vi "Replace Array Subset (Multi).vi"(5 "JSON Array":refnum<class "JSON Array.lvclass">, 9 "index":i32, 11 "new element/subarray":refnum<class "JSON Null.lvclass">[](array[class])) -> (6 "output JSON Array":refnum<class "JSON Array.lvclass">)   [LabVIEW 2016, in "LVJSON.lvlib" / "JSON Array.lvclass"]
doc: "Replaces an element or subarray in an array at the point you specify in index."
uses:
  JSON Array.lvclass
  JSON Datatype/JSON Null.lvclass
  JSON Array.lvclass/JSON Array.ctl
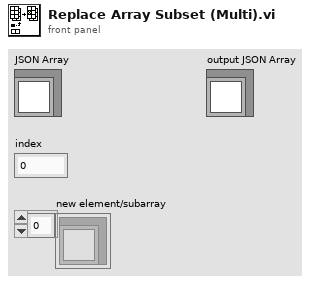
[diagram p1: front panel]
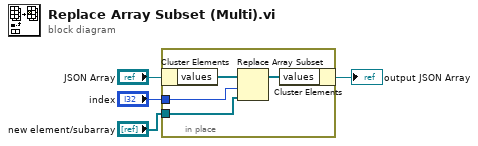
[diagram p0: block diagram]
diagram:
  n1 = in-place {
    in-place-border: "new element/subarray" -> [w8]
    in-place-border: "index" -> [w7]
    n2 = in-place-cluster #1("JSON Array") -> ("values"=w6:refnum<class "JSON Null.lvclass">[])
    n3 = Replace Array Subset(array=w6, new element=w8, index=w7) -> (w5:refnum<class "JSON Null.lvclass">[])
    n4 = in-place-cluster #1("values"=w5) -> (→"output JSON Array":refnum<class "JSON Array.lvclass">)
  }
